vi "Target_9.vi"   [LabVIEW 2023]
uses:
  <vilib>/Platform/TimedLoop/XDataNode/timing_clust.ctl
  <vilib>/Platform/TimedLoop/XDataNode/nitl_modes.ctl
  <vilib>/Platform/TimedLoop/XDataNode/wakeup.ctl
  <vilib>/Platform/TimedLoop/XDataNode/XDataNode.xnode
  <vilib>/Platform/TimedLoop/XDataNode/XDNodeRunTimeDep.lvlib
  <vilib>/measure/NI_MABase.lvlib
types:
  T1 = typedef "XDNodeRunTimeDep.lvlib/timing_clust.ctl" = cluster{"Expected End [f-1]":u64, "Actual End [f-1]":u64, "Finished Late? [f-1]":bool, "Expected End [i-1]":u64, "Actual End [i-1]":u64, "Finished Late? [i-1]":bool, "Expected Start [i]":u64, "Actual Start [i]":u64, "Expected Start [f]":u64, "Actual Start [f]":u64, "Source Name":string, "Structure Name":string, "Period":i64, "Deadline":i64, "Offset":i64, "Start":i64, "Priority":i32, "Timeout":i32, "Mode":T2, "Wakeup Reason":T3, "Error":errorcluster, "Source Type":string, "Secondary Source Type":string, "Global End Time":u64, "Global Start Time":u64, "Frame Duration":u64, "Iteration Duration":u64, "Assigned CPU":i32, "I/O Scan Engine Mode":u32}
  T2 = typedef "XDNodeRunTimeDep.lvlib/nitl_modes.ctl" = enum32{"No Change", "Process missed periods, maintain original phase", "Discard missed periods, maintain original phase", "Process missed periods, ignore original phase", "Discard missed periods, ignore original phase"}
  T3 = typedef "XDNodeRunTimeDep.lvlib/wakeup.ctl" = enum32{"Normal", "Aborted", "Asynchronous wakeup", "Timing source error", "Timed loop error", "Timeout"}
  T4 = enum16{"Sine Wave", "Triangle Wave", "Square Wave", "Sawtooth Wave"}
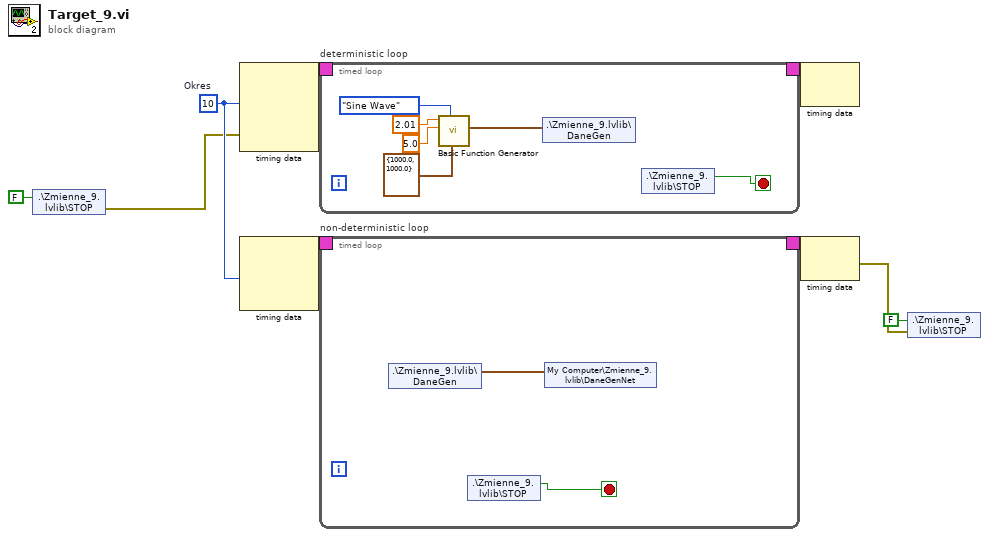
[diagram p0: block diagram]
diagram:
  w5 = i64 10  # Okres
  n1 = shared-variable ".\\Zmienne_9.lvlib\\STOP"(FALSE ("STOP")) -> (error out=w3:errorcluster)  [unwired: 1 in]
  n2 = node-c288 ("Input Node")(w5, w3) -> (w9:T1)  [unwired: 2 in]
  n3 = node-c288 ("Input Node")(w5) -> (w7:T1)  [unwired: 2 in]
  n4 = timed-loop "deterministic loop" {
    timing: w9 -> [_]
    timing-out: [_] -> w8
    stop <- w10 stop-if-true
    n5 = call <vilib>:"Basic Function Generator.vi"("sampling info"=cluster{"Fs":dbl, "#s":dbl} {"Fs"=1000.0, "#s"=1000.0}, "signal type"=T4."Sine Wave", "amplitude"=5.0, "frequency"=2.01) -> ("signal out"=w11:waveform(dbl))  [unwired: 5 in, 2 out]
    n6 = shared-variable ".\\Zmienne_9.lvlib\\DaneGen"(w11) -> ()  [unwired: 1 in, 1 out]
    n7 = shared-variable ".\\Zmienne_9.lvlib\\STOP"() -> (w10:bool)  [unwired: 1 in, 1 out]
  }
  n8 = timed-loop "non-deterministic loop" {
    timing: w7 -> [_]
    timing-out: [_] -> w6
    stop <- w19 stop-if-true
    n9 = shared-variable ".\\Zmienne_9.lvlib\\DaneGen"() -> (w18:waveform(dbl))  [unwired: 1 in, 1 out]
    n10 = shared-variable ".\\Zmienne_9.lvlib\\STOP"() -> (w19:bool)  [unwired: 1 in, 1 out]
    n11 = shared-variable "My Computer\\Zmienne_9.lvlib\\DaneGenNet"(w18) -> ()  [unwired: 1 in, 1 out]
  }
  n12 = node-c288 ("Output Node")(w8) -> ()  [unwired: 1 out]
  n13 = node-c288 ("Output Node")(w6) -> (w1:errorcluster)
  n14 = shared-variable ".\\Zmienne_9.lvlib\\STOP"(FALSE ("STOP"), error in=w1) -> ()  [unwired: 1 out]
